vi "Get Type.vi"(11 "I32 in":refnum<class "I32.lvclass">) -> (3 "Type":string)   [LabVIEW 2020, in "I32.lvclass"]
uses:
  <vilib>/gpm_packages/@cs/data-type-serializer/source/I32/I32.lvclass
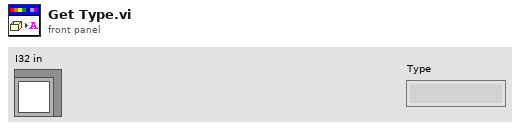
[diagram p1: front panel]
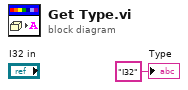
[diagram p0: block diagram]
diagram:
  "Type" <- "I32" ("Type")
